vi "test_definitions_module.vi"(6 "Delay":dbl min=0.0 format="%.2f", 7 "Mode":T2(ring), 8 "error in (no error)":errorcluster, 10 "VISA resource in 19572":refnum<visa-resource-name>="COM6", 11 "VISA resource in 19052":refnum<visa-resource-name>="COM5") -> (0 "error out":errorcluster, 3 "Mode parameters":T1 {"Total test time" format="%.2f"; "overlap" format="%.2f"; "Second time test" format="%.2f"; "First time test" format="%.2f"})   [LabVIEW 2015]
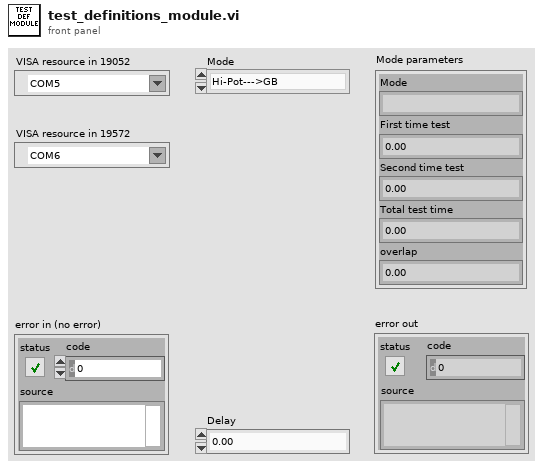
[diagram p1: front panel]
types:
  T1 = cluster{"First time test":dbl, "Second time test":dbl, "overlap":dbl, "Total test time":dbl, "Mode":string}
  T2 = enum16{"Hi-Pot--->GB", "GB--->Hi-Pot", "Hi-Pot only", "GB only"}
  T3 = cluster{"steps":u16[], "times":string[], "active steps":u16, "modes":string[], "Total time":dbl, "CONT.?":bool}
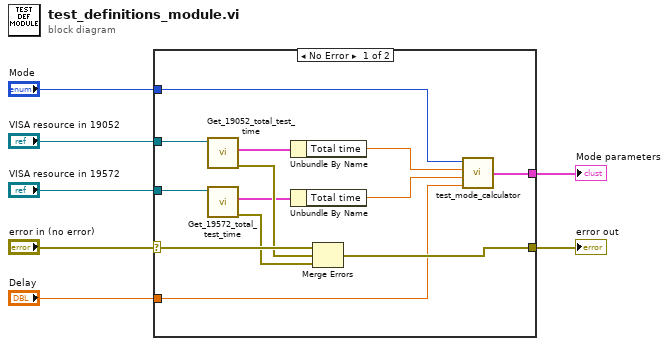
[diagram p0: block diagram]
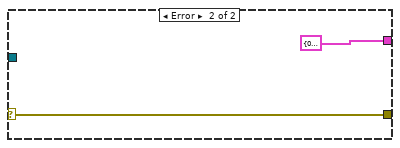
[diagram p2: hidden frame]
diagram:
  n1 = case shown="No Error" "error in (no error)" {
    selector: "error in (no error)" -> [w20 w22]
    tunnel: "VISA resource in 19052" -> [w19 _]
    tunnel: "VISA resource in 19572" -> [w10 _]
    tunnel: [w18 w22] -> w5
    tunnel: "Mode" -> [w15 _]
    tunnel: "Delay" -> [w12 _]
    tunnel: [w11 T1 {"First time test"=0.0, "Second time test"=0.0, "overlap"=0.0, "Total test time"=0.0, "Mode"=""} ("Mode parameters")] -> w2
    frame No Error {
      n2 = call "Get_19052_total_test_time.vi"("VISA resource in"=w19) -> ("error out"=w16:errorcluster, "Data"=w8:T3)  [unwired: 8 in, 1 out]
      n3 = call "Get_19572_total_test_time.vi"("VISA resource in"=w10) -> ("error out"=w17:errorcluster, "Data"=w9:T3)  [unwired: 8 in, 1 out]
      n4 = Unbundle By Name(w8) -> ("Total time"=w14:dbl)
      n5 = Unbundle By Name(w9) -> ("Total time"=w13:dbl)
      n6 = Merge Errors(w20, w16, w17) -> (w18:errorcluster)
      n7 = call "test_mode_calculator.vi"("Mode"=w15, "T1"=w14, "Delay"=w13, "T2"=w12) -> ("Mode parameters"=w11:T1)  [unwired: 3 in]
    }
    frame Error {
    }
  }
  "error out" <- w5
  "Mode parameters" <- w2
